vi "Untitled 1.vi"() -> ()   [LabVIEW 2015]
panel:
  in  "stop":bool
  in  "back":bool
  out "Сдача":u8
  out "Picture":i32(slide) scale=0.0..10.0
  in  "cancel":bool
  out "Недостаточно \n     средств":bool
  in  "С сиропом?":bool
  in  "Газированая?":bool
  in  "Fill":bool
  out "Сумма средств":u8
  in  "coin":enum16{"5 рублей", "10 рублей"}(ring)
  in  "Enum":enum16{"water", "gas", "syrup", "odd", "stop"}(ring)
  in  "enter":bool
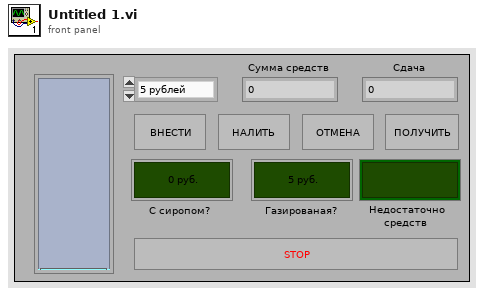
[diagram p1: front panel]
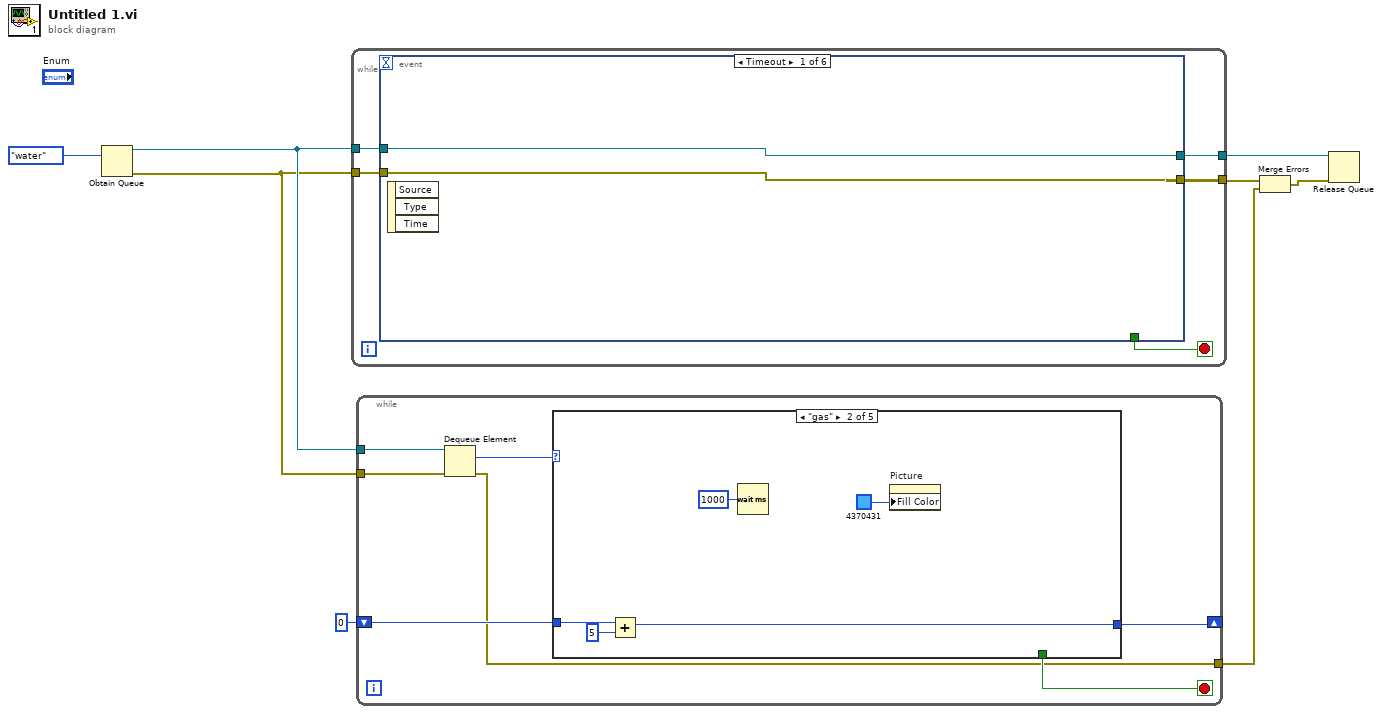
[diagram p0: block diagram]
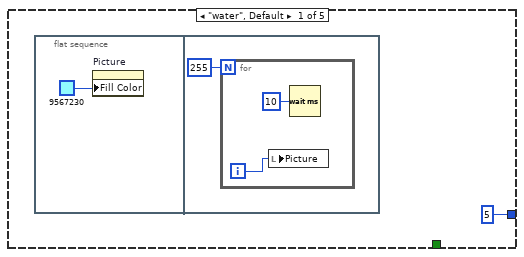
[diagram p2: hidden frame]
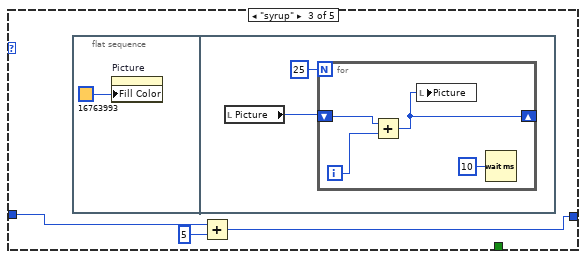
[diagram p3: hidden frame]
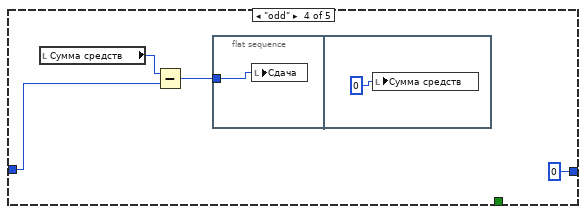
[diagram p4: hidden frame]
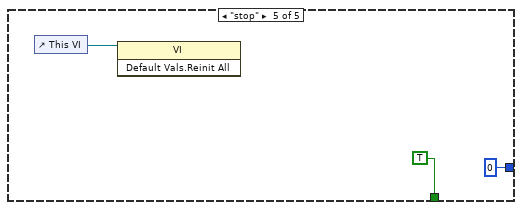
[diagram p5: hidden frame]
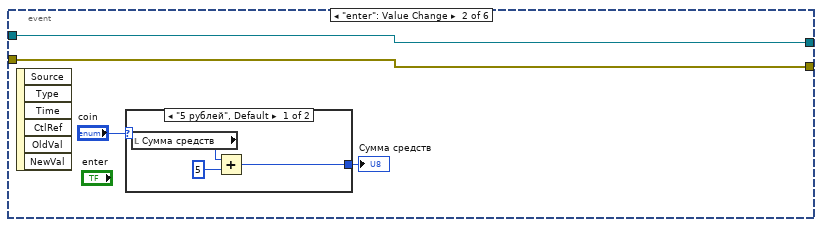
[diagram p6: hidden frame]
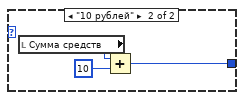
[diagram p7: hidden frame]
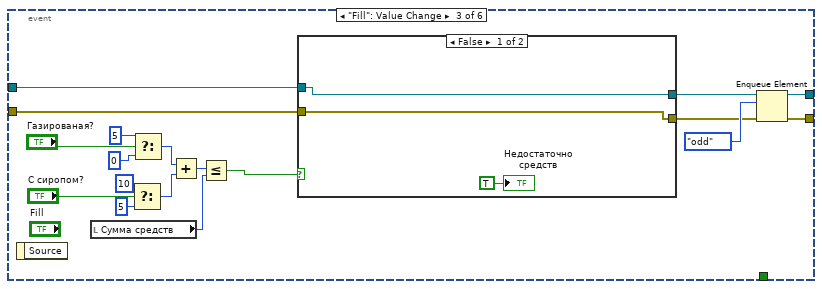
[diagram p8: hidden frame]
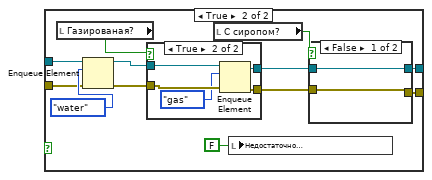
[diagram p9: hidden frame]
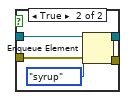
[diagram p10: hidden frame]
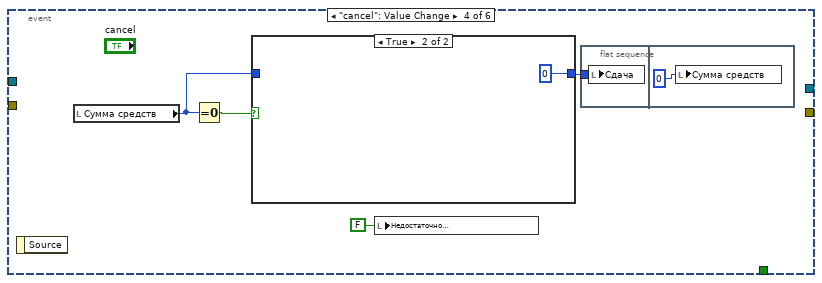
[diagram p12: hidden frame]
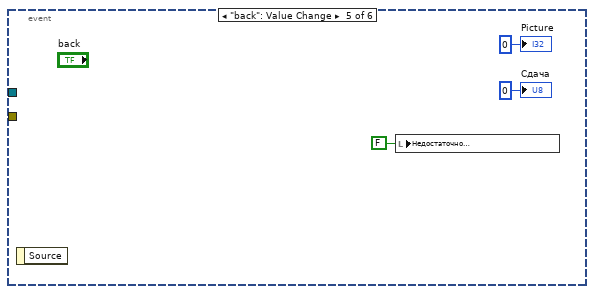
[diagram p14: hidden frame]
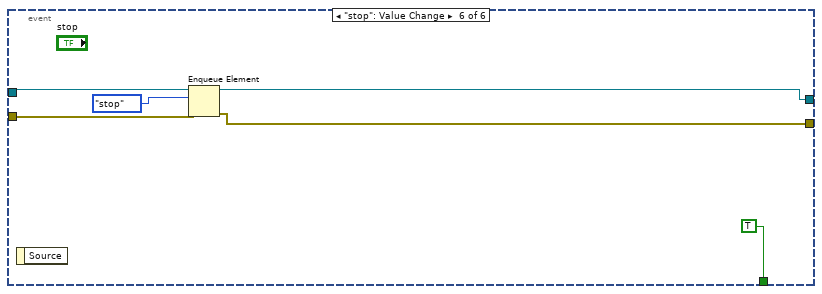
[diagram p15: hidden frame]
diagram:
  n1 = Obtain Queue(element data type=enum16{"water", "gas", "syrup", "odd", "stop"}."water" ("Enum")) -> (queue out=w4:refnum<queue>, error out=w3:errorcluster)  [unwired: 4 in, 1 out]
  n2 = while {
    tunnel: w4 -> [w13]
    tunnel: w3 -> [w12]
    tunnel: [w11] -> w6
    tunnel: [w10] -> w7
    stop <- w9 stop-if-true
    n3 = event shown="[0] Timeout" {
      selector: _ -> [_ _ _ _ _ _]
      dyn-events: _ -> [_ _ _ _ _ _]
      timeout: _ -> [_ _ _ _ _ _]
      tunnel: w13 -> [w15 w17 w30 _ _ w87]
      tunnel: w12 -> [w14 w16 w29 _ _ w86]
      tunnel: [w15 w17 w31 _ _ w85] -> w11
      tunnel: [w14 w16 w32 _ _ w84] -> w10
      tunnel: [_ _ _ _ _ TRUE] -> w9
      event Timeout {
        n4 = event-data() -> ()  [unwired: 1 in, 3 out]
      }
      event "enter": Value Change {
        n5 = event-data() -> ()  [unwired: 1 in, 6 out]
        n6 = case shown="\"5 рублей\", Default" "coin" {
          tunnel: [w20 w23] -> w18
          frame "5 рублей", Default {
            n7 = local read "Сумма средств"() -> (w22:u8)
            n8 = Add(x=w22, y=u8 5) -> (x+y=w20:u8)
          }
          frame "10 рублей" {
            n9 = local read "Сумма средств"() -> (w25:u8)
            n10 = Add(x=w25, y=u8 10) -> (x+y=w23:u8)
          }
        }
        "Сумма средств" <- w18
      }
      event "Fill": Value Change {
        n11 = event-data() -> ()  [unwired: 1 in, 1 out]
        n12 = local read "Сумма средств"() -> (w34:u8)
        n13 = Select(t=u8 10, s="С сиропом?", f=u8 5) -> (s? t:f=w36:u8)
        n14 = Select(t=u8 5, s="Газированая?", f=u8 0) -> (s? t:f=w37:u8)
        n15 = Add(x=w37, y=w36) -> (x+y=w35:u8)
        n16 = Less Or Equal?(x=w35, y=w34) -> (x <= y?=w33:bool)
        n17 = case shown="False" w33 {
          tunnel: w30 -> [w45 w57]
          tunnel: w29 -> [w44 w56]
          tunnel: [w45 w48] -> w27
          tunnel: [w44 w49] -> w26
          frame False {
            "Недостаточно \n     средств" <- TRUE ("Недостаточно \n     средств")
          }
          frame True {
            n18 = local read "Газированая?"() -> (w55:bool)
            n19 = Enqueue Element(queue=w57, element=enum16{"water", "gas", "syrup", "odd", "stop"}."water" ("Enum"), error in (no error)=w56) -> (queue out=w54:refnum<queue>, error out=w53:errorcluster)  [unwired: 1 in, 1 out]
            n20 = case shown="True" w55 {
              tunnel: w54 -> [w67 w72]
              tunnel: w53 -> [w66 w71]
              tunnel: [w66 w69] -> w51
              tunnel: [w67 w68] -> w50
              frame False {
              }
              frame True {
                n21 = Enqueue Element(queue=w72, element=enum16{"water", "gas", "syrup", "odd", "stop"}."gas" ("Enum"), error in (no error)=w71) -> (queue out=w68:refnum<queue>, error out=w69:errorcluster)  [unwired: 1 in, 1 out]
              }
            }
            n22 = local read "С сиропом?"() -> (w52:bool)
            n23 = local write "Недостаточно \n     средств"(FALSE ("Недостаточно \n     средств")) -> ()
            n24 = case shown="False" w52 {
              tunnel: w51 -> [w59 w64]
              tunnel: w50 -> [w60 w63]
              tunnel: [w59 w61] -> w49
              tunnel: [w60 w62] -> w48
              frame False {
              }
              frame True {
                n25 = Enqueue Element(queue=w63, element=enum16{"water", "gas", "syrup", "odd", "stop"}."syrup" ("Enum"), error in (no error)=w64) -> (queue out=w62:refnum<queue>, error out=w61:errorcluster)  [unwired: 1 in, 1 out]
              }
            }
          }
        }
        n26 = Enqueue Element(queue=w27, element=enum16{"water", "gas", "syrup", "odd", "stop"}."odd" ("Enum"), error in (no error)=w26) -> (queue out=w31:refnum<queue>, error out=w32:errorcluster)  [unwired: 1 in, 1 out]
      }
      event "cancel": Value Change {
        n27 = event-data() -> ()  [unwired: 1 in, 1 out]
        n28 = local read "Сумма средств"() -> (w74:u8)
        n29 = Equal To 0?(x=w74) -> (x = 0?=w76:bool)
        n30 = case shown="True" w76 {
          tunnel: [w79 u8 0 ("Сдача")] -> w75
          tunnel: w74 -> [w79 _]
          frame False {
          }
          frame True {
          }
        }
        n31 = local write "Недостаточно \n     средств"(FALSE ("Недостаточно \n     средств")) -> ()
        n32 = flat-sequence {
          tunnel: w75 -> [w77]
          frame #0 {
            n33 = local write "Сдача"(w77) -> ()
          }
          frame #1 {
            n34 = local write "Сумма средств"(u8 0 ("Сумма средств")) -> ()
          }
        }
      }
      event "back": Value Change {
        n35 = event-data() -> ()  [unwired: 1 in, 1 out]
        n36 = local write "Недостаточно \n     средств"(FALSE ("Недостаточно \n     средств")) -> ()
        "Picture" <- 0 ("Picture")
        "Сдача" <- u8 0 ("Сдача")
      }
      event "stop": Value Change {
        n37 = event-data() -> ()  [unwired: 1 in, 1 out]
        n38 = Enqueue Element(queue=w87, element=enum16{"water", "gas", "syrup", "odd", "stop"}."stop" ("Enum"), error in (no error)=w86) -> (queue out=w85:refnum<queue>, error out=w84:errorcluster)  [unwired: 1 in, 1 out]
      }
    }
  }
  n39 = while {
    tunnel: w4 -> [w96]
    tunnel: w3 -> [w95]
    shift-right: [w93] -> _
    shift-left: u8 0 -> [w92]
    tunnel: [w90] -> w1
    stop <- w91 stop-if-true
    n40 = Dequeue Element(queue=w96, error in (no error)=w95) -> (element=w94:enum16{"water", "gas", "syrup", "odd", "stop"}, error out=w90:errorcluster)  [unwired: 1 in, 2 out]
    n41 = case shown="\"gas\"" w94 {
      tunnel: [u8 5 w102 w107 u8 0 u8 0] -> w93
      tunnel: w92 -> [_ w104 w109 w119 _]
      tunnel: [_ _ _ _ TRUE] -> w91
      frame "water", Default {
        n42 = flat-sequence {
          frame #0 {
            n43 = property on="Picture" class="Slide (strict)"("Fill Color"=u32 9567230) -> ()  [unwired: 2 in, 2 out]
          }
          frame #1 {
            n44 = for {
              N: 255 -> [_]
              i -> [w101]
              n45 = local write "Picture"(w101) -> ()
              n46 = Wait (ms)(milliseconds to wait=u32 10) -> ()  [unwired: 1 out]
            }
          }
        }
      }
      frame "gas" {
        n47 = Add(x=w104, y=u8 5) -> (x+y=w102:u8)
        n48 = Wait (ms)(milliseconds to wait=u32 1000) -> ()  [unwired: 1 out]
        n49 = property on="Picture" class="Slide (strict)"("Fill Color"=u32 4370431) -> ()  [unwired: 2 in, 2 out]
      }
      frame "syrup" {
        n50 = flat-sequence {
          frame #0 {
            n51 = property on="Picture" class="Slide (strict)"("Fill Color"=u32 16763993) -> ()  [unwired: 2 in, 2 out]
          }
          frame #1 {
            n52 = local read "Picture"() -> (w111:i32)
            n53 = for {
              N: 25 -> [_]
              shift-right: [w113] -> _
              shift-left: w111 -> [w115]
              i -> [w114]
              n54 = Add(x=w115, y=w114) -> (x+y=w113:i32)
              n55 = local write "Picture"(w113) -> ()
              n56 = Wait (ms)(milliseconds to wait=u32 10) -> ()  [unwired: 1 out]
            }
          }
        }
        n57 = Add(x=w109, y=u8 5) -> (x+y=w107:u8)
      }
      frame "odd" {
        n58 = local read "Сумма средств"() -> (w120:u8)
        n59 = Subtract(x=w120, y=w119) -> (x-y=w118:u8)
        n60 = flat-sequence {
          tunnel: w118 -> [w121]
          frame #0 {
            n61 = local write "Сдача"(w121) -> ()
          }
          frame #1 {
            n62 = local write "Сумма средств"(u8 0 ("Сумма средств")) -> ()
          }
        }
      }
      frame "stop" {
        n63 = control-ref of="This VI"() -> (w123:refnum<vi>)
        n64 = invoke class="VI" method="Default Vals.Reinit All"(reference=w123) -> ()  [unwired: 2 in, 3 out]
      }
    }
  }
  n65 = Merge Errors(w7, w1) -> (w8:errorcluster)
  n66 = Release Queue(queue=w6, error in (no error)=w8) -> ()  [unwired: 1 in, 3 out]
